vi "Close.vi"(8 "error in":errorcluster, 11 "Tool Tip Text in":refnum<class "Tool Tip Text.lvclass">) -> (0 "error out":errorcluster, 3 "Tool Tip Text out":refnum<class "Tool Tip Text.lvclass">)   [LabVIEW 2023, in "SourceGrid.lvlib" / "Tool Tip Text.lvclass"]
uses:
  Tool Tip Text.lvclass
  Tool Tip Text.lvclass/Tool Tip Text.ctl
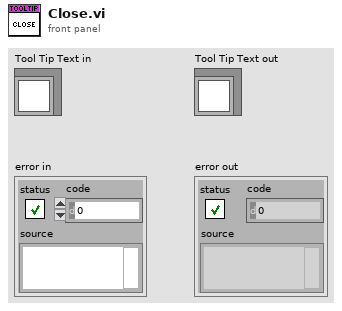
[diagram p1: front panel]
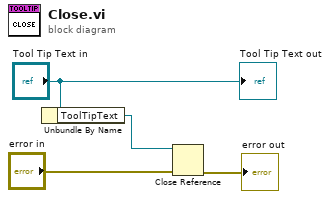
[diagram p0: block diagram]
diagram:
  n1 = Unbundle By Name("Tool Tip Text in") -> ("ToolTipText"=w1:refnum<k24>)
  n2 = Close Reference(reference=w1, error in (no error)="error in") -> (error out=→"error out":errorcluster)
  "Tool Tip Text out" <- "Tool Tip Text in"
